vi "Thermocouple-ContinuousInput.vi"() -> ()   [LabVIEW 2016]
doc: "This example demonstrates how to continuously acquire temperature measurements using a DAQmx device.\n\nFor instructions on how to connect your signals to the DAQ device, refer to your device documentation."
uses:
  <vilib>/Utility/error.llb/DialogType.ctl
  <vilib>/DAQmx/read.llb/DAQmx Read (Analog 1D Wfm NChan NSamp).vi
  <vilib>/DAQmx/create/channels.llb/DAQmx Create Channel (AI-Temperature-Thermocouple).vi
  <vilib>/DAQmx/configure/timing.llb/DAQmx Timing (Sample Clock).vi
  <vilib>/DAQmx/configure/trigger.llb/DAQmx Start Trigger (Digital Edge).vi
  <vilib>/DAQmx/configure/trigger.llb/DAQmx Start Trigger (Analog Edge).vi
  <vilib>/DAQmx/miscellaneous.llb/DAQmx Fill In Error Info.vi
  <resource>/objmgr/daqmx.rc
panel:
  in  "Trigger Type":T1(tab)
  in  "Digital Start Trigger Edge":i32(ring)=10280 caption="Edge" items=["Rising"=10280, "Falling"=10171]
  in  "Digital Start Trigger Source":tag="/Dev1/PFI0" caption="Source"
  in  "Digital Pause Trigger Pause When":i32(ring)=10192 caption="Pause When" items=["High"=10192, "Low"=10214]
  in  "Digital Pause Trigger Source":tag="/Dev1/PFI0" caption="Source"
  in  "Analog Start Trigger Level":dbl caption="Level" format="%0.2f"
  in  "Analog Start Trigger Hysteresis":dbl caption="Hysteresis" format="%.2f"
  in  "Analog Start Trigger Slope":i32(ring)=10280 caption="Slope" items=["Rising"=10280, "Falling"=10171]
  in  "Analog Start Trigger Source":string="APFI0" caption="Source"
  in  "Analog Pause Trigger Source":string="APFI0" caption="Source"
  in  "Analog Pause Trigger Pause When":i32(ring)=10093 caption="Pause When" items=["Above Level"=10093, "Below Level"=10107]
  in  "Analog Pause Trigger Level":dbl caption="Level" format="%.2f"
  in  "CJC Source":i32(ring)=10116 items=["Built-In"=10200, "Constant Value"=10116, "Channel"=10113]
  in  "Thermocouple Type":i32(ring)=10072 items=["J"=10072, "K"=10073, "N"=10077, "R"=10082, "S"=10085, "T"=10086, "B"=10047, "E"=10055]
  in  "Enable Autozero":bool caption="Enable\nAutozero*"
  in  "Auto Zero Mode":i32(ring)=10230 items=["None"=10230, "Once"=10244, "Every Sample"=10164]
  in  "CJC Channel":refnum<k21>
  in  "CJC Value (deg C)":dbl=25.0 format="%0.2f"
  in  "Stop":bool
  out "Waveform Graph":waveform(dbl)[](graph)
  in  "Samples per Loop":i32=100
  in  "Sample Rate":dbl=1000.0
  in  "Sample Clock Source":tag="OnboardClock"
  in  "Max Value (deg C)":dbl=100.0
  in  "Min Value (deg C)":dbl
  in  "Physical Channel":tag="Dev1/ai0"
  out "Actual Sample Rate":dbl format="%0.2f"
  # "Channel Settings"
  # "Acquired Data"
  # "High Accuracy Settings"
  # "* Some devices do not support Auto Zero Mode."
  # "Trigger Settings"
  # "Timing Settings"
  # "To enable triggers, select a tab above, and configure the settings.\n\nNot all hardware supports all trigger types. Refer to your device documentation for more information."
  # "This trigger type is not supported in continuous sample timing. \n\nRefer to your device documentation for more information on which triggers are supported."
  # "This trigger type is not supported in continuous sample timing. \n\nRefer to your device documentation for more information on which triggers are supported."
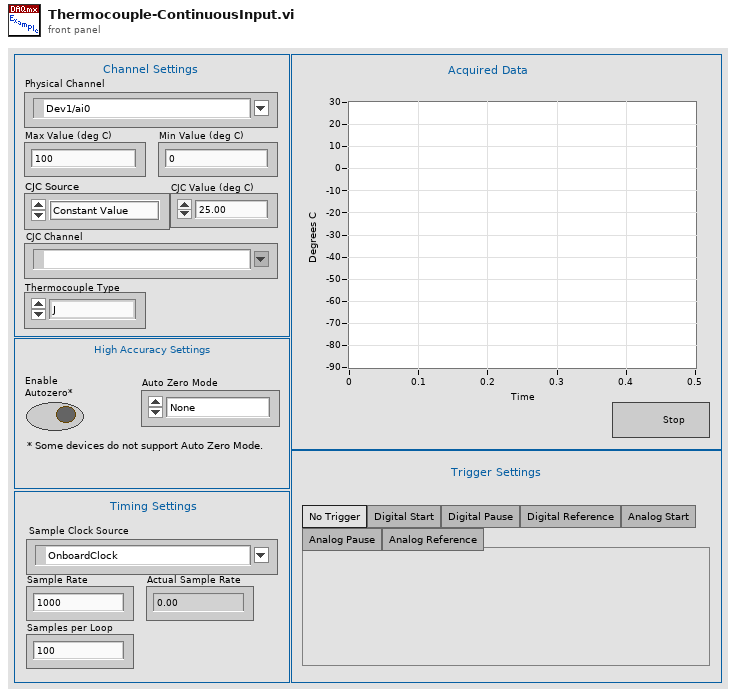
[diagram p1: front panel]
types:
  T1 = enum32{"No Trigger", "Digital Start", "Digital Pause", "Digital Reference", "Analog Start", "Analog Pause", "Analog Reference"}
  T2 = typedef "DialogType.ctl" = u16
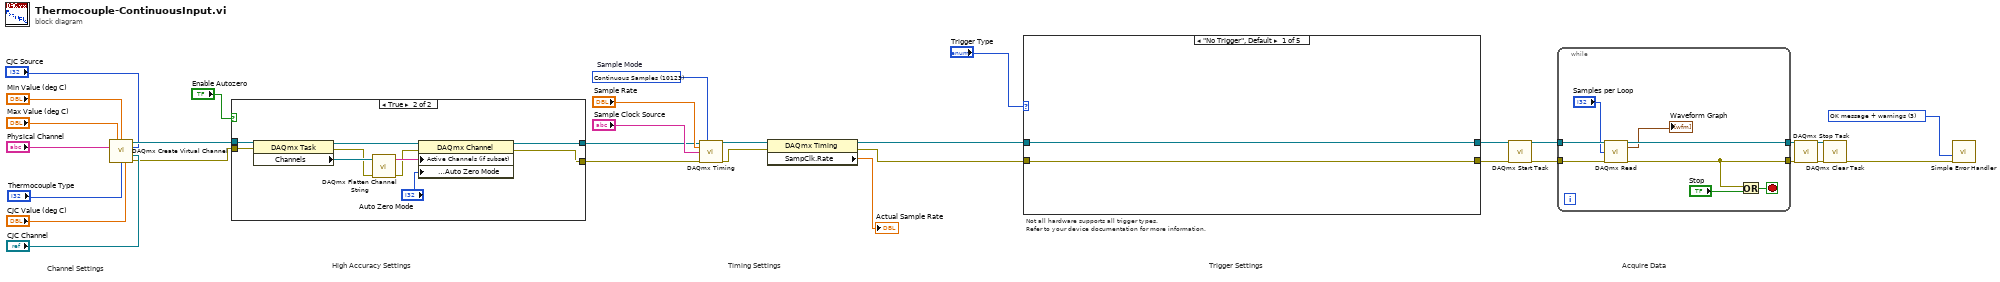
[diagram p0: block diagram]
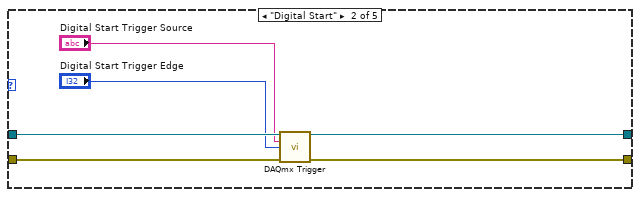
[diagram p2: hidden frame]
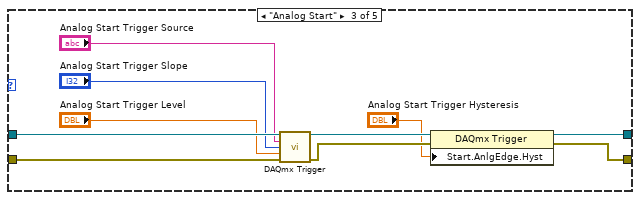
[diagram p3: hidden frame]
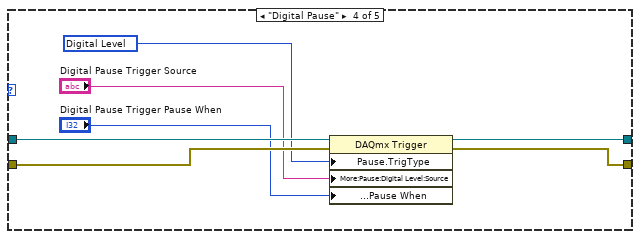
[diagram p4: hidden frame]
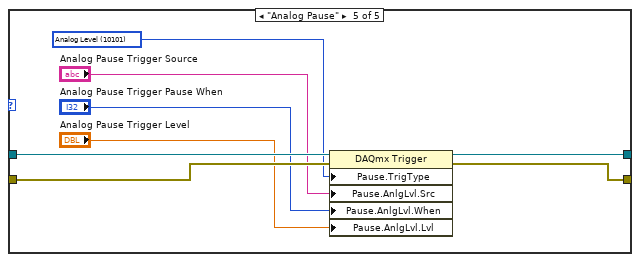
[diagram p5: hidden frame]
diagram:
  w6 = T2 3 items=["no dialog", "OK message", "continue or stop message", "OK message + warnings", "continue/stop + warnings"] ("type of dialog (OK msg:1)")
  w29 = 10123 items=["Finite Samples"=10178, "Continuous Samples"=10123, "Hardware Timed Single Point"=12522]  # Sample Mode
  # "Trigger Settings"
  # "Not all hardware supports all trigger types.\nRefer to your device documentation for more information."
  # "High Accuracy Settings"
  # "Acquire Data"
  # "Timing Settings"
  # "Channel Settings"
  n1 = call-poly <vilib>:"DAQmx Create Virtual Channel.vi"("maximum value"="Max Value (deg C)", "minimum value"="Min Value (deg C)", "physical channels"="Physical Channel", "cjc source"="CJC Source", "cjc channel"="CJC Channel", "thermocouple type"="Thermocouple Type", "cjc value"="CJC Value (deg C)") -> ("task out"=w17:refnum<k21>, "error out"=w16:errorcluster)  [unwired: 7 in]
  n2 = case shown="True" "Enable Autozero" {
    tunnel: w17 -> [w32 w42]
    tunnel: w16 -> [w33 w41]
    tunnel: [w32 w37] -> w14
    tunnel: [w33 w36] -> w13
    frame False {
      # "Bypass Auto-Zero"
    }
    frame True {
      n3 = property class="DAQmx Task"(reference=w42, error in=w41) -> (reference out=w40:refnum<k21>, error out=w35:errorcluster, "Channels"=w39:refnum<k21>[])
      n4 = call <vilib>:"DAQmx Flatten Channel String.vi"("names in"=w39, "error in"=w35) -> ("names out"=w38:string, "error out"=w34:errorcluster)  [unwired: 12 in]
      n5 = property class="DAQmx Channel"(reference=w40, error in=w34, "Active Channels (if subset)"=w38, "Analog Input:General Properties:Advanced:High Accuracy Settings:Auto Zero Mode"="Auto Zero Mode") -> (reference out=w37:refnum<k21>, error out=w36:errorcluster)
    }
  }
  n6 = call-poly <vilib>:"DAQmx Timing.vi"("task/channels in"=w14, "sample mode"=w29, "rate"="Sample Rate", "source"="Sample Clock Source", "error in"=w13) -> ("task out"=w31:refnum<k21>, "error out"=w30:errorcluster)  [unwired: 9 in]
  n7 = property class="DAQmx Timing"(reference=w31, error in=w30) -> (reference out=w3:refnum<k21>, error out=w4:errorcluster, "SampClk.Rate"=→"Actual Sample Rate":dbl)
  n8 = case shown="\"No Trigger\", Default" "Trigger Type" {
    tunnel: w3 -> [w45 w51 w61 w68 w76]
    tunnel: w4 -> [w44 w50 w60 w65 w73]
    tunnel: [w45 w49 w58 w67 w75] -> w1
    tunnel: [w44 w48 w57 w66 w74] -> w2
    frame "No Trigger", Default {
    }
    frame "Digital Start" {
      n9 = call-poly <vilib>:"DAQmx Trigger.vi"("task/channels in"=w51, "source"="Digital Start Trigger Source", "edge"="Digital Start Trigger Edge", "error in"=w50) -> ("task out"=w49:refnum<k21>, "error out"=w48:errorcluster)  [unwired: 10 in]
    }
    frame "Analog Start" {
      n10 = call-poly <vilib>:"DAQmx Trigger.vi"("task/channels in"=w61, "source"="Analog Start Trigger Source", "slope"="Analog Start Trigger Slope", "level"="Analog Start Trigger Level", "error in"=w60) -> ("task out"=w56:refnum<k21>, "error out"=w55:errorcluster)  [unwired: 9 in]
      n11 = property class="DAQmx Trigger"(reference=w56, error in=w55, "Start.AnlgEdge.Hyst"="Analog Start Trigger Hysteresis") -> (reference out=w58:refnum<k21>, error out=w57:errorcluster)
    }
    frame "Digital Pause" {
      w64 = 10152 items=["Analog Level"=10101, "Analog Window"=10103, "Digital Level"=10152, "Digital Pattern"=10398, "None"=10230] ("Pause.TrigType")
      n12 = property class="DAQmx Trigger"(reference=w68, error in=w65, "Pause.TrigType"=w64, "More:Pause:Digital Level:Source"="Digital Pause Trigger Source", "More:Pause:Digital Level:Pause When"="Digital Pause Trigger Pause When") -> (reference out=w67:refnum<k21>, error out=w66:errorcluster)
    }
    frame "Analog Pause" {
      w72 = 10101 items=["Analog Level"=10101, "Analog Window"=10103, "Digital Level"=10152, "Digital Pattern"=10398, "None"=10230] ("Pause.TrigType")
      n13 = property class="DAQmx Trigger"(reference=w76, error in=w73, "Pause.TrigType"=w72, "Pause.AnlgLvl.Src"="Analog Pause Trigger Source", "Pause.AnlgLvl.When"="Analog Pause Trigger Pause When", "Pause.AnlgLvl.Lvl"="Analog Pause Trigger Level") -> (reference out=w75:refnum<k21>, error out=w74:errorcluster)
    }
  }
  n14 = call <vilib>:"DAQmx Start Task.vi"("task/channels in"=w1, "error in"=w2) -> ("task out"=w28:refnum<k21>, "error out"=w27:errorcluster)  [unwired: 12 in]
  n15 = while {
    tunnel: w28 -> [w84]
    tunnel: w27 -> [w83]
    tunnel: [w77] -> w7
    tunnel: [w81] -> w8
    stop <- w82 stop-if-true
    n16 = call-poly <vilib>:"DAQmx Read.vi"("task/channels in"=w84, "number of samples per channel"="Samples per Loop", "error in"=w83) -> ("task out"=w81:refnum<k21>, "data"=→"Waveform Graph":waveform(dbl)[], "error out"=w77:errorcluster)  [unwired: 10 in]
    n17 = Or(x=w77, y="Stop") -> (x .or. y?=w82:bool)
  }
  n18 = call <vilib>:"DAQmx Stop Task.vi"("task/channels in"=w8, "error in"=w7) -> ("task out"=w10:refnum<k21>, "error out"=w9:errorcluster)  [unwired: 12 in]
  n19 = call <vilib>:"DAQmx Clear Task.vi"("task in"=w10, "error in"=w9) -> ("error out"=w26:errorcluster)  [unwired: 13 in]
  n20 = call <vilib>:"Simple Error Handler.vi"("type of dialog (OK msg:1)"=w6, "error in (no error)"=w26) -> ()  [unwired: 3 in, 5 out]
